vi "Set Trigger Parameters.vi"(7 "DG Number":i32, 8 "error in (no error)":errorcluster, 11 "Settings":T1={"T Delay (µs)"=0.0, "T Set Back"=1.0, "T Triggers"=1, "T Active"=TRUE, "T Polarity"=TRUE, "T Term"=FALSE, "T Drive"=FALSE, "A Delay (µs)"=3.0, "A Set Back"=1.0, "A Triggers"=1, "A Active"=TRUE, "A Polarity"=TRUE, "A Term"=FALSE, "A Drive"=FALSE, "B Delay (µs)"=4.0, "B Set Back"=1.0, "B Triggers"=1, "B Active"=TRUE, "B Polarity"=TRUE, "B Term"=FALSE, "B Drive"=FALSE, "Gate A*B"=FALSE, "Output\nLevel"=1, "Trigger\nTerminate"=TRUE, "Clock\nEnable"=TRUE, "Internal\nClock (µs)"=1.0, "Trigger\nLevel"=10.0, "Stop\nTrigger"=1, "Ocillator\nDivide By"=1, "Clock Source"=1, "Gate Divider"=1, "Positive\nGate"=TRUE, "Trigger\nSource"=FALSE, "Internal\nArming"=FALSE, "Software\nTrigger"=TRUE, "Trigger\nSlope"=FALSE, "Stop on\nPreset"=TRUE, "Trigger\nOperation"=TRUE, "Trigger\nEnable"=TRUE} {"B Set Back" min=0.0 format="%.3f"; "A Set Back" min=0.0 format="%.3f"; "T Set Back" min=0.0 format="%.3f"; "Clock Source" items=["Internal Oscillator"=1, "External Trigger"=2, "Trigger & Oscillator"=3, "Master Slave Bus"=4]; "Trigger\nLevel" min=0.0 format="%.3f"; "Output\nLevel" items=["TTL"=1, "NIM"=2, "ECL"=3]; "Internal\nClock (µs)" min=0.0 format="%.4f"; "B Delay (µs)" min=0.0 format="%.3f"; "A Delay (µs)" min=0.0 format="%.3f"; "T Delay (µs)" min=0.0 format="%.3f"}) -> (0 "error out":errorcluster)   [LabVIEW 2009, in "POLARIS BME DG.lvlib"]
doc: "long Set_TriggerParameters(BOOL TriggerTerminate, double InternalClock, double TriggerLevel, unsigned long PresetValue, unsigned long GateDivider, BOOL PositiveGate, BOOL InternalTrigger, BOOL InternalArm, BOOL SoftwareTrigger, BOOL RisingEdge, BOOL StopOnPreset, BOOL ResetWhenDone, BOOL TriggerEnable, long DG_Number);"
uses:
  POLARIS BME DG.lvlib
  Settings.ctl
  BME DLL/DelayGenerator.dll
panel:
  # "NOTICE -- YOU MUST LEAVE THIS NOTICE IN PLACE.  PER THE TERMS OF THE LICENSE BELOW, YOU MAY SUBLICENSE THIS SOFTWARE \nIN ANY WAY THAT DOES NOT CONFLICT WITH THIS LICENSE.\n\n### BSD License (http://www.opensource.org/licenses/bsd-license.php) Begin ###\n \nCopyright (c) 2011, Applied Energetics, http://www.appliedenergetics.com,\n                               Richard Schwerdtfeger, <rschwerdtfeger@appliedenergetics.com>\n\nAll rights reserved.\n\nRedistribution and use in source and binary forms, with or without modification, are permitted provided that the \nfollowing conditions are met:\n\n    * Redistributions of source code must retain the above copyright notice, this list of conditions and the following disclaimer.\n    * Redistributions in binary form must reproduce the above copyright notice, this list of conditions and the following disclaimer \n       in the documentation and/or other materials provided with the distribution.\n    * Neither the name of Richard Schwerdtfeger, Applied Energetics, Inc., nor the names of its contributors may be used to \n       endorse or promote products derived from this software without specific prior written permission.\n\nTHIS SOFTWARE IS PROVIDED BY THE COPYRIGHT HOLDERS AND CONTRIBUTORS \"AS IS\" AND ANY EXPRESS OR IMPLIED WARRANTIES, \nINCLUDING, BUT NOT LIMITED TO, THE IMPLIED WARRANTIES OF MERCHANTABILITY AND FITNESS FOR A PARTICULAR PURPOSE ARE \nDISCLAIMED. IN NO EVENT SHALL THE COPYRIGHT OWNER OR CONTRIBUTORS BE LIABLE FOR ANY DIRECT, INDIRECT, INCIDENTAL,\n SPECIAL, EXEMPLARY, OR CONSEQUENTIAL DAMAGES (INCLUDING, BUT NOT LIMITED TO, PROCUREMENT OF SUBSTITUTE GOODS OR \nSERVICES; LOSS OF USE, DATA, OR PROFITS; OR BUSINESS INTERRUPTION) HOWEVER CAUSED AND ON ANY THEORY OF LIABILITY, \nWHETHER IN CONTRACT, STRICT LIABILITY, OR TORT (INCLUDING NEGLIGENCE OR OTHERWISE) ARISING IN ANY WAY OUT OF THE USE \nOF THIS SOFTWARE, EVEN IF ADVISED OF THE POSSIBILITY OF SUCH DAMAGE.\n\n### BSD License End ###"
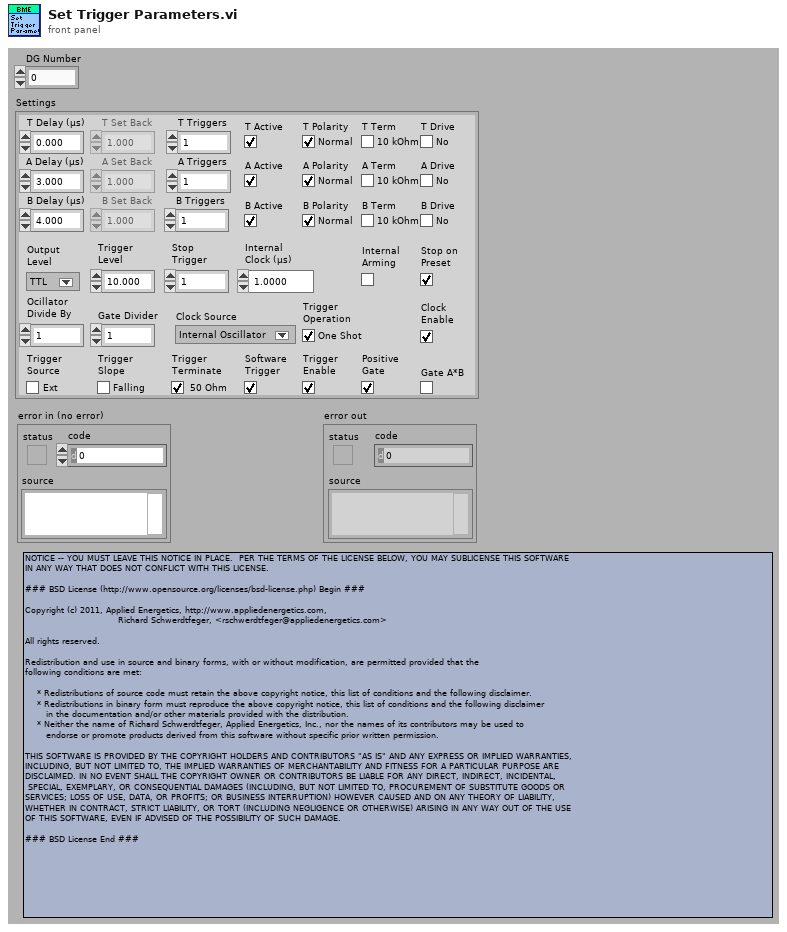
[diagram p1: front panel]
types:
  T1 = typedef "POLARIS BME DG.lvlib/Settings.ctl" = cluster{"T Delay (µs)":dbl, "T Set Back":dbl, "T Triggers":u16, "T Active":bool, "T Polarity":bool, "T Term":bool, "T Drive":bool, "A Delay (µs)":dbl, "A Set Back":dbl, "A Triggers":u16, "A Active":bool, "A Polarity":bool, "A Term":bool, "A Drive":bool, "B Delay (µs)":dbl, "B Set Back":dbl, "B Triggers":u16, "B Active":bool, "B Polarity":bool, "B Term":bool, "B Drive":bool, "Gate A*B":bool, "Output\nLevel":u32, "Trigger\nTerminate":bool, "Clock\nEnable":bool, "Internal\nClock (µs)":dbl, "Trigger\nLevel":dbl, "Stop\nTrigger":u32, "Ocillator\nDivide By":u16, "Clock Source":u32, "Gate Divider":u32, "Positive\nGate":bool, "Trigger\nSource":bool, "Internal\nArming":bool, "Software\nTrigger":bool, "Trigger\nSlope":bool, "Stop on\nPreset":bool, "Trigger\nOperation":bool, "Trigger\nEnable":bool}
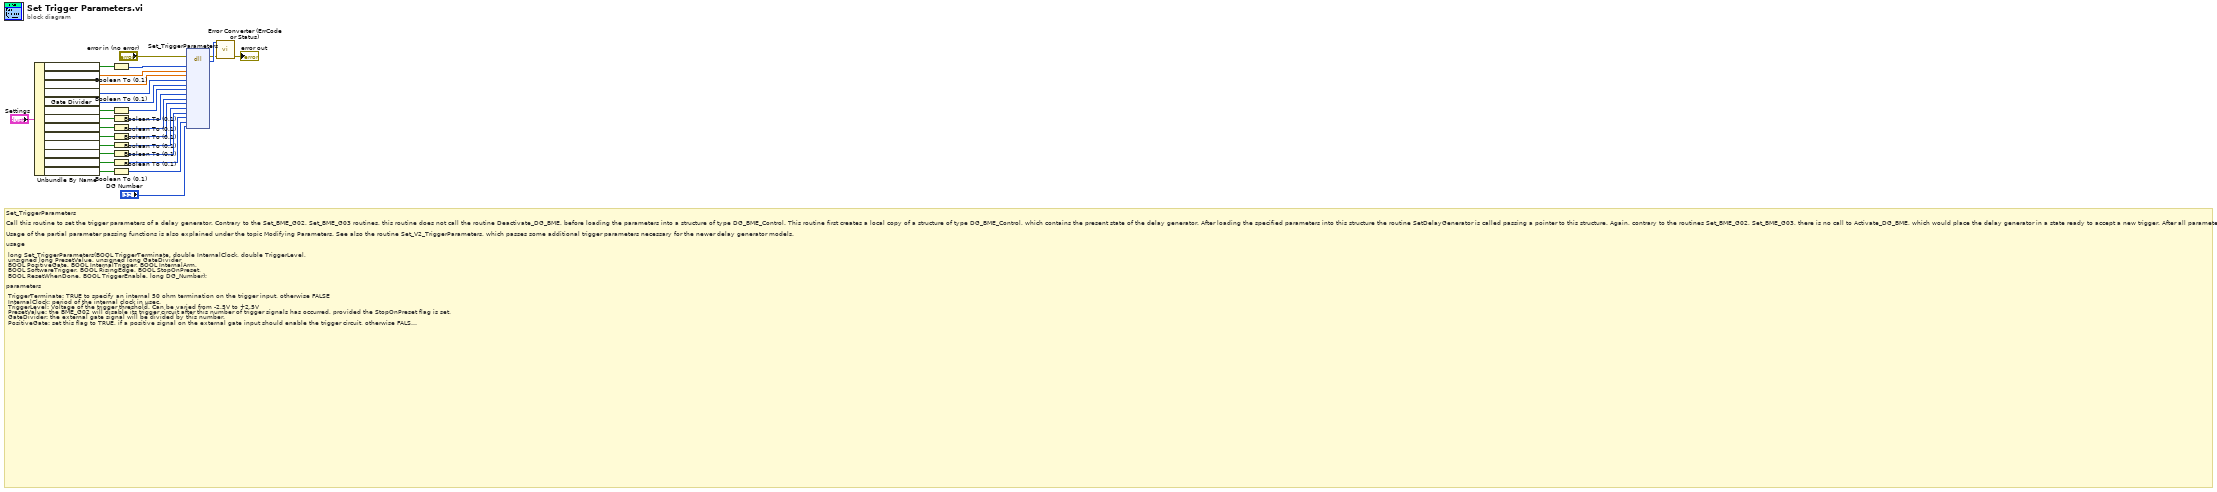
[diagram p0: block diagram]
diagram:
  # "Set_TriggerParameters\n\nCall this routine to set the trigger parameters of a delay generator. Contrary to the Set_BME_G02, Set_BME_G03 routines, this routine does not call the routine Deactivate_DG_BME, before loading the parameters into a structure of type DG_BME_Control. This routine first creates a local copy of a structure of type DG_BME_Control, which contains the present state of the delay generator. After loading the specified parameters into this structure the routine SetDelayGenerator is called passing a pointer to this structure. Again, contrary to the routines Set_BME_G02, Set_BME_G03, there is no call to Activate_DG_BME, which would place the delay generator in a state ready to accept a new trigger. After all parameters have been loaded, an explicit call to Activate_DG_BME is necessary.\n\nUsage of the partial parameter passing functions is also explained under the topic Modifying Parameters. See also the routine Set_V2_TriggerParameters, which passes some additional trigger parameters necessary for the newer delay generator models.\n\nusage\n\n long Set_TriggerParameters(BOOL TriggerTerminate, double InternalClock, double TriggerLevel,\n unsigned long PresetValue, unsigned long GateDivider\n BOOL PositiveGate, BOOL InternalTrigger, BOOL InternalArm,\n BOOL SoftwareTrigger, BOOL RisingEdge, BOOL StopOnPreset,\n BOOL ResetWhenDone, BOOL TriggerEnable, long DG_Number);\n\nparameters\n\n TriggerTerminate: TRUE to specify an internal 50 ohm termination on the trigger input, otherwise FALSE\n InternalClock: period of the internal clock in µsec.\n TriggerLevel: Voltage of the trigger threshold. Can be varied from -2.5V to +2.5V\n PresetValue: the BME_G02 will disable its trigger circuit after this number of trigger signals has occurred, provided the StopOnPreset flag is set.\n GateDivider: the external gate signal will be divided by this number.\n PositiveGate: set this flag to TRUE, if a positive signal on the external gate input should enable the trigger circuit, otherwise FALSE. Note that the TriggerEnable flag is or’ed with the external gate signal. Only when the TriggerEnable flag is set FALSE, the trigger circuit can be enabled by the external gate signal.\n InternalTrigger: if this flag is set the BME_G02 will be triggered by its internal clock, (provided it is jumpered as a master module).\n InternalArm: if this flag is set the external trigger of the BME_G02 will be armed by its internal clock, (provided it is jumpered as a master module).\n SoftwareTrigger: if this flag is set the BME_G02 will be triggered by the SoftwareTrigger_DG_BME routine, (provided it is jumpered as a master module). The flags InternalTrigger and SoftwareTrigger may not be set at the same time.\n RisingEdge: if none of the flags InternalTrigger or SoftwareTrigger are set and this module is jumpered as master, the BME_G02 will be triggered by the rising edge of a signal applied to its external connector.\n StopOnPreset: if this flag is set, the BME_G02 will disable its trigger circuit when the number of triggers prescribed by PresetValue has been reached. Modules slaved to a master will also stop at this point.\n ResetWhenDone: if this flag is set, all outputs from master and slave(s) will be reset to their untriggered states 2 µsec after the last delay of master and slave(s) has elapsed. This function is controlled by the master module. If this flag is not set, all modules, master and slave(s) have to be individually reset by calling the two routines Deactivate_DG_BME and Activate_DG_BME (in that order).\n TriggerEnable: this flag must be set to enable the trigger circuit. This signal is or'ed with the signal coming from the external gate input. Actually, the rising edge of the (divided) gate signal clocks a flip-flop allowing a trigger. After a trigger has occurred, the flip-flop is reset.\n DG_Number: The number of the delay generator as assigned by the\n\nInitialize_DG_BME routine\n\nreturn value\n\n 0: success\n 2: DG_Number is out of range"
  n1 = Unbundle By Name("Settings") -> ("Trigger\nTerminate"=w22:bool, "Internal\nClock (µs)"=w20:dbl, "Trigger\nLevel"=w19:dbl, "Stop\nTrigger"=w18:u32, "Gate Divider"=w17:u32, "Positive\nGate"=w16:bool, "Trigger\nSource"=w14:bool, "Internal\nArming"=w11:bool, "Software\nTrigger"=w12:bool, "Trigger\nSlope"=w8:bool, "Stop on\nPreset"=w6:bool, "Trigger\nOperation"=w5:bool, "Trigger\nEnable"=w2:bool)
  n2 = Boolean To (0,1)(Boolean=w22) -> (0, 1=w21:i16)
  n3 = Boolean To (0,1)(Boolean=w16) -> (0, 1=w15:i16)
  n4 = Boolean To (0,1)(Boolean=w14) -> (0, 1=w13:i16)
  n5 = Boolean To (0,1)(Boolean=w11) -> (0, 1=w10:i16)
  n6 = Boolean To (0,1)(Boolean=w12) -> (0, 1=w9:i16)
  n7 = Boolean To (0,1)(Boolean=w8) -> (0, 1=w7:i16)
  n8 = Boolean To (0,1)(Boolean=w6) -> (0, 1=w4:i16)
  n9 = Boolean To (0,1)(Boolean=w5) -> (0, 1=w3:i16)
  n10 = Boolean To (0,1)(Boolean=w2) -> (0, 1=w1:i16)
  n11 = dll-call lib="C:/CS Framework/LVSCC/LV2009/GPL/Projects/cs-framework/CSClass/CSPOLARIS/POLARIS BME DG/BME DLL/DelayGenerator.*" fn="Set_TriggerParameters"(error in="error in (no error)", "TriggerTerminate"=w21, "InternalClock"=w20, "TriggerLevel"=w19, "PresetValue"=w18, "GateDivider"=w17, "PositiveGate"=w15, "InternalTrigger"=w13, "InternalArm"=w10, "SoftwareTrigger"=w9, "RisingEdge"=w7, "StopOnPreset"=w4, "ResetWhenDone"=w3, "TriggerEnable"=w1, "DG_Number"="DG Number") -> (error out=w25:errorcluster, "return type"=w28:i32)  [unwired: 16 in, 1 out]
  n12 = call "Error Converter (ErrCode or Status).vi"("error in (no error)"=w25, "error code"=w28) -> ("error out"=→"error out":errorcluster)  [unwired: 9 out]
